vi "Write Switch Heater.vi"(8 "error in (no error)":errorcluster, 10 "Turn SH On?":bool, 11 "Power Supply in":refnum<class "Power Supply.lvclass">) -> (0 "error out":errorcluster, 3 "Power Supply out":refnum<class "Power Supply.lvclass">)   [LabVIEW 2009, in "Power Supply.lvclass"]
uses:
  Power Supply.lvclass
  Switch Heater Status.ctl
  Power Supply.lvclass/Power Supply.ctl
panel:
  in  "interrupt":bool
  out "done":bool
  out "busybar":bool[](array[boolean])
  out "time":string
  out "display":string
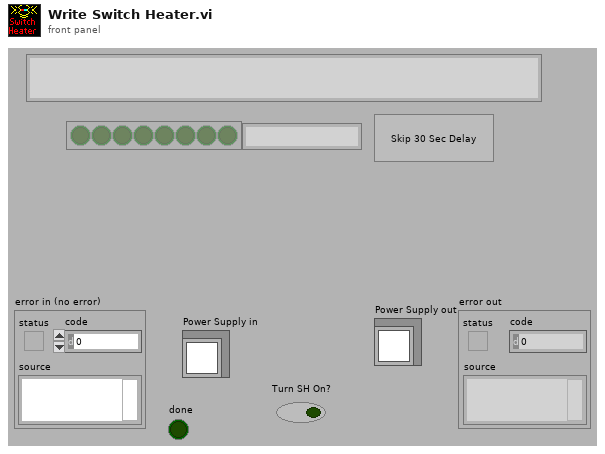
[diagram p1: front panel]
types:
  T1 = typedef "Power Supply.lvclass/Switch Heater Status.ctl" = enum16{"Off (at zero)", "On", "Off (at field)", "Other"}
  T2 = typedef "PSIO.ctl" = cluster{"Address":T3, "Version":enum16{"PS", "IPS"}}
  T3 = typedef "OxfordAddress.ctl" = cluster{"Com Port":i32, "ISOBUS Address":i32, "GPIB Address":i16, "Communication":enum16{"RS232", "ISOBUS", "GPIB", "Gateway"}}
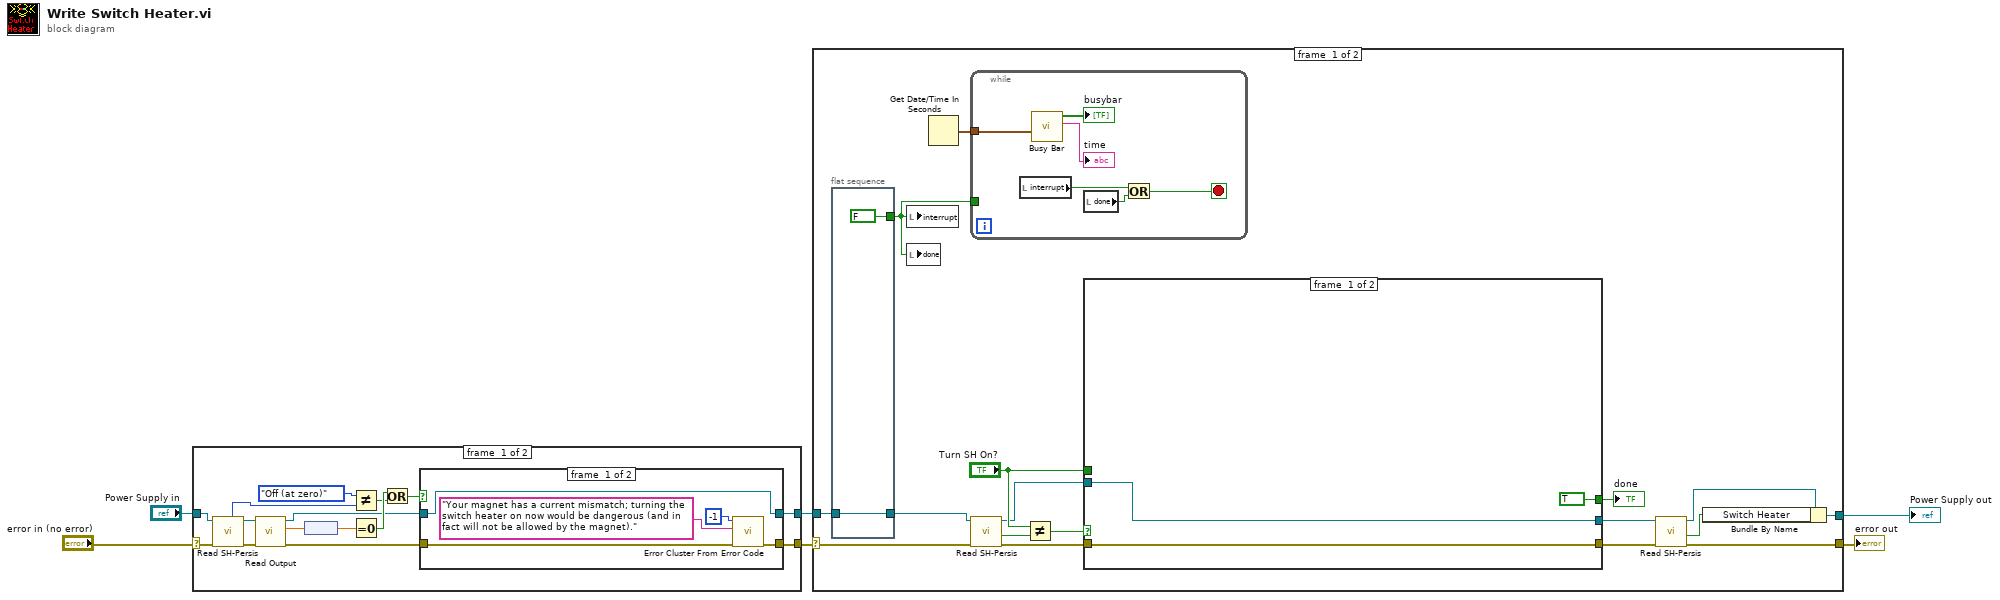
[diagram p0: block diagram]
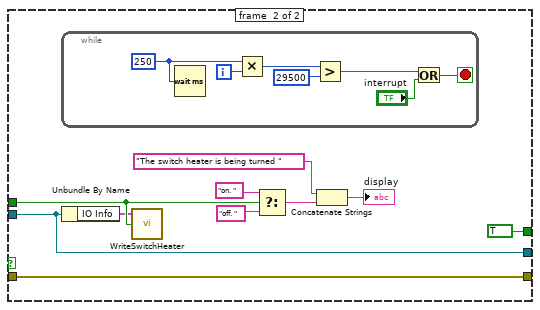
[diagram p4: hidden frame]
diagram:
  n1 = case shown="No Error" "error in (no error)" {
    selector: "error in (no error)" -> [w10 w29]
    tunnel: [w13 w30] -> w4
    tunnel: [w12 w29] -> w3
    tunnel: "Power Supply in" -> [w11 w30]
    frame #0 {
      n2 = call-dynamic "Read SH-Persis.vi"("error in (no error)"=w10, "Power Supply in"=w11) -> ("error out"=w17:errorcluster, "Power Supply out"=w16:refnum<class "Power Supply.lvclass">, "SHstatus"=w9:T1)  [unwired: 4 in, 3 out]
      n3 = call-dynamic "Read Output.vi"("error in (no error)"=w17, "Power Supply in"=w16) -> ("error out"=w18:errorcluster, "Field"=w19:dbl[unit], "Power Supply out"=w15:refnum<class "Power Supply.lvclass">)  [unwired: 6 in, 1 out]
      n4 = node(w19) -> (w14:dbl)
      n5 = Not Equal?(x=Switch_Heater_Status."Off (at zero)", y=w9) -> (x != y?=w7:bool)
      n6 = Equal To 0?(x=w14) -> (x = 0?=w21:bool)
      n7 = Or(x=w21, y=w7) -> (x .or. y?=w20:bool)
      n8 = case shown="False" w20 {
        tunnel: w18 -> [w25 w28]
        tunnel: w15 -> [w26 w27]
        tunnel: [w26 w27] -> w13
        tunnel: [w24 w28] -> w12
        frame #0 {
          n9 = call <vilib>:"Error Cluster From Error Code.vi"("error in (no error)"=w25, "error message (\"\")"="Your magnet has a current mismatch; turning the switch heater on now would be dangerous (and in fact will not be allowed by the magnet).", "error code (0)"=-1) -> ("error out"=w24:errorcluster)  [unwired: 6 in]
        }
        frame #1 {
        }
      }
    }
    frame #1 {
    }
  }
  n10 = case shown="Error" w3 {
    selector: w3 -> [w44 w76]
    tunnel: w4 -> [w47 w77]
    tunnel: [w46 w77] -> w6
    tunnel: [w45 w76] -> w5
    frame #0 {
      n11 = flat-sequence {
        tunnel: w47 -> [w75]
        tunnel: [w75] -> w43
        tunnel: [FALSE] -> w31
        frame #0 {
        }
      }
      n12 = local write "interrupt"(w31) -> ()
      n13 = local write "done"(w31) -> ()
      n14 = Get Date/Time In Seconds() -> (seconds since 1Jan1904=w42:timestamp)
      n15 = while {
        tunnel: w42 -> [w68]
        tunnel: w31 -> [_]
        stop <- w71 stop-if-true
        n16 = local read "interrupt"() -> (w69:bool)
        n17 = call "Busy Bar.vi"("basetime"=w68) -> ("Time"=→"time":string, "Busy Bar"=→"busybar":bool[])  [unwired: 1 in, 8 out]
        n18 = local read "done"() -> (w70:bool)
        n19 = Or(x=w69, y=w70) -> (x .or. y?=w71:bool)
      }
      n20 = call-dynamic "Read SH-Persis.vi"("error in (no error)"=w44, "Power Supply in"=w43) -> ("error out"=w35:errorcluster, "SHon?"=w37:bool, "Power Supply out"=w36:refnum<class "Power Supply.lvclass">)  [unwired: 4 in, 3 out]
      n21 = Not Equal?(x="Turn SH On?", y=w37) -> (x != y?=w39:bool)
      n22 = case shown="True" w39 {
        tunnel: "Turn SH On?" -> [_ w60]
        tunnel: [w50 w54] -> w41
        tunnel: w36 -> [w50 w54]
        tunnel: w35 -> [w49 w52]
        tunnel: [w49 w52] -> w40
        tunnel: [TRUE TRUE] -> w34
        frame #0 {
        }
        frame #1 {
          n23 = while {
            i -> [w66]
            stop <- w67 stop-if-true
            w65 = 250
            n24 = Wait (ms)(milliseconds to wait=w65) -> ()  [unwired: 1 out]
            n25 = Multiply(x=w65, y=w66) -> (x*y=w64:i32)
            n26 = Greater?(x=w64, y=29500) -> (0:w63:bool)
            n27 = Or(x=w63, y="interrupt") -> (x .or. y?=w67:bool)
          }
          n28 = Unbundle By Name(w54) -> ("IO Info"=w53:T2)
          n29 = call "WriteSwitchHeater.vi"("Switch Heater On"=w60, "IO Info"=w53) -> ()  [unwired: 1 in, 2 out]
          n30 = Select(t="on. ", s=w60, f="off. ") -> (s? t:f=w56:string)
          n31 = Concatenate Strings("The switch heater is being turned ", w56) -> (→"display":string)
        }
      }
      "done" <- w34
      n32 = call-dynamic "Read SH-Persis.vi"("error in (no error)"=w40, "Power Supply in"=w41) -> ("error out"=w45:errorcluster, "SHon?"=w32:bool, "Power Supply out"=w33:refnum<class "Power Supply.lvclass">)  [unwired: 4 in, 3 out]
      n33 = Bundle By Name(cluster=w33, "Switch Heater"=w32) -> (w46:refnum<class "Power Supply.lvclass">)
    }
    frame #1 {
    }
  }
  "error out" <- w5
  "Power Supply out" <- w6
